vi "Process State Buffer.vi"(2 "AccelGyro constants":T3={"gyrRange"=0.0, "accRange"=0.0, "gx offset"=0.0, "gy offset"=0.0, "gz offset"=0.0, "ax offset"=0.0, "ay offset"=0.0, "az offset"=0.0, "axyz scale"=1.0} {"axyz scale" format="%#_4f"; "az offset" format="%#_4f"; "ay offset" format="%#_4f"; "ax offset" format="%#_4f"; "gz offset" format="%#_4f"; "gy offset" format="%#_4f"; "gx offset" format="%#_4f"; "gyrRange" format="%#_4f"; "accRange" format="%#_4f"}, 3 "STATE_Buffer excluding '$' [1...30]":string) -> (0 "Inertial state values":T2 {"w_z (dps)" format="%#_4f"; "a_y (g)" format="%#_4f"; "a_z (g)" format="%#_4f"; "w_y (dps)" format="%#_4f"; "a_x (g)" format="%#_4f"; "Sensor temp. (degC)" format="%#.2f"; "w_x (dps)" format="%#_4f"}, 1 "Environmental state values":T1 {"Dew point (degC)" format="%#.2f"; "Density (kg/m^3)" format="%#.3f"; "Pressure alt. (m)" format="%#.2f"; "Density alt. (m)" format="%#.2f"; "Rel. Humidity (%)" format="%#.2f"; "P_atmos (Pa)" format="%#_6f"; "Sensor temp. (degC)" format="%#.2f"; "Thermistor (degC)" format="%#.2f"})   [LabVIEW 2020]
uses:
  Ctls/AccelGyro constants.ctl
  Ctls/Inertial state values.ctl
  Ctls/Environmental state values.ctl
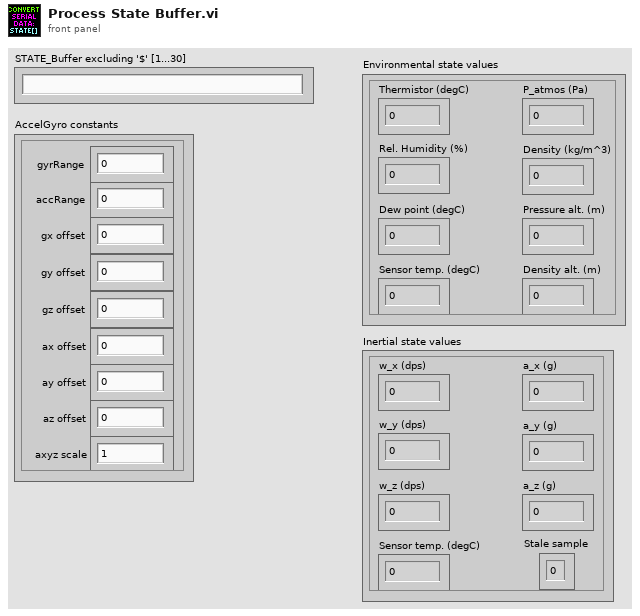
[diagram p1: front panel]
types:
  T1 = typedef "Environmental state values.ctl" = cluster{"Thermistor (degC)":sgl, "Sensor temp. (degC)":sgl, "P_atmos (Pa)":sgl, "Rel. Humidity (%)":sgl, "Density (kg/m^3)":sgl, "Dew point (degC)":sgl, "Pressure alt. (m)":sgl, "Density alt. (m)":sgl}
  T2 = typedef "Inertial state values.ctl" = cluster{"w_x (dps)":sgl, "w_y (dps)":sgl, "w_z (dps)":sgl, "a_x (g)":sgl, "a_y (g)":sgl, "a_z (g)":sgl, "Stale sample":u8, "Sensor temp. (degC)":sgl}
  T3 = typedef "AccelGyro constants.ctl" = cluster{"gyrRange":sgl, "accRange":sgl, "gx offset":sgl, "gy offset":sgl, "gz offset":sgl, "ax offset":sgl, "ay offset":sgl, "az offset":sgl, "axyz scale":sgl}
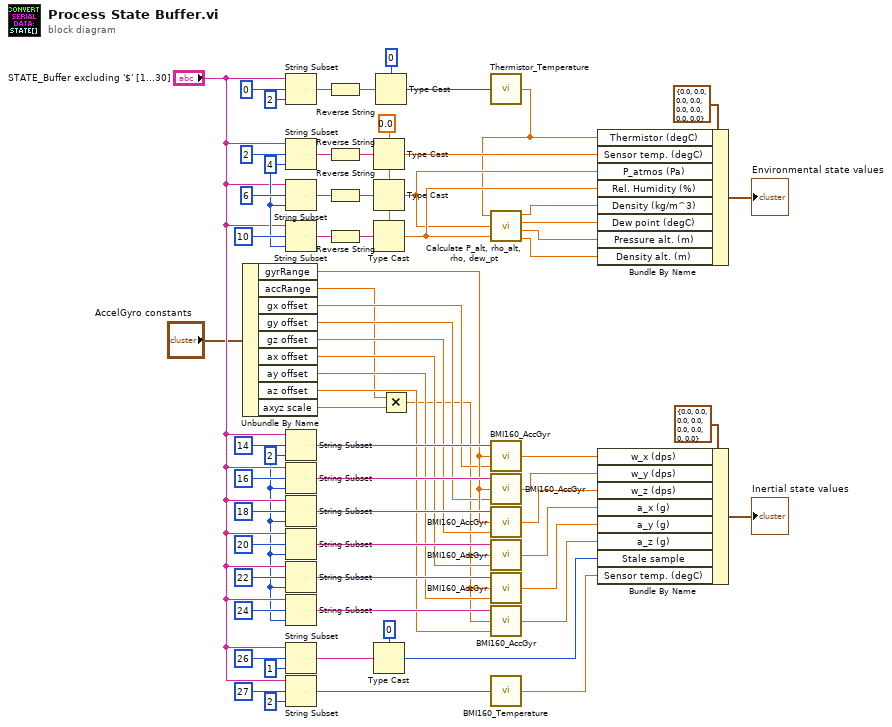
[diagram p0: block diagram]
diagram:
  w38 = 2 ("length (rest)")
  w58 = sgl 0.0
  w56 = 4 ("length (rest)")
  n1 = Unbundle By Name("AccelGyro constants") -> ("gyrRange"=w36:sgl, "accRange"=w28:sgl, "gx offset"=w35:sgl, "gy offset"=w34:sgl, "gz offset"=w33:sgl, "ax offset"=w32:sgl, "ay offset"=w31:sgl, "az offset"=w30:sgl, "axyz scale"=w29:sgl)
  n2 = String Subset(string="STATE_Buffer excluding '$' [1...30]", offset (0)=0, length (rest)=2 ("length (rest)")) -> (substring=w67:string)
  n3 = String Subset(string="STATE_Buffer excluding '$' [1...30]", offset (0)=2, length (rest)=w56) -> (substring=w63:string)
  n4 = String Subset(string="STATE_Buffer excluding '$' [1...30]", offset (0)=6, length (rest)=w56) -> (substring=w62:string)
  n5 = String Subset(string="STATE_Buffer excluding '$' [1...30]", offset (0)=10, length (rest)=w56) -> (substring=w59:string)
  n6 = String Subset(string="STATE_Buffer excluding '$' [1...30]", offset (0)=14, length (rest)=w38) -> (substring=w55:string)
  n7 = String Subset(string="STATE_Buffer excluding '$' [1...30]", offset (0)=16, length (rest)=w38) -> (substring=w54:string)
  n8 = String Subset(string="STATE_Buffer excluding '$' [1...30]", offset (0)=18, length (rest)=w38) -> (substring=w50:string)
  n9 = String Subset(string="STATE_Buffer excluding '$' [1...30]", offset (0)=20, length (rest)=w38) -> (substring=w51:string)
  n10 = String Subset(string="STATE_Buffer excluding '$' [1...30]", offset (0)=22, length (rest)=w38) -> (substring=w47:string)
  n11 = String Subset(string="STATE_Buffer excluding '$' [1...30]", offset (0)=24, length (rest)=w38) -> (substring=w46:string)
  n12 = String Subset(string="STATE_Buffer excluding '$' [1...30]", offset (0)=26, length (rest)=1 ("length (rest)")) -> (substring=w42:string)
  n13 = String Subset(string="STATE_Buffer excluding '$' [1...30]", offset (0)=27, length (rest)=2 ("length (rest)")) -> (substring=w37:string)
  n14 = Reverse String(1:w67) -> (0:w13:string)
  n15 = Reverse String(1:w63) -> (0:w12:string)
  n16 = Reverse String(1:w62) -> (0:w11:string)
  n17 = Reverse String(1:w59) -> (0:w10:string)
  n18 = Type Cast(type=w58, x=w12) -> (*(type *) &x=w3:sgl)
  n19 = Type Cast(type=w58, x=w11) -> (*(type *) &x=w4:sgl)
  n20 = Type Cast(type=w58, x=w10) -> (*(type *) &x=w5:sgl)
  n21 = Type Cast(type=u8 0, x=w42) -> (*(type *) &x=w17:u8)
  n22 = Type Cast(type=u16 0, x=w13) -> (*(type *) &x=w65:u16)
  n23 = Multiply(x=w28, y=w29) -> (x*y=w27:sgl)
  n24 = call "Thermistor_Temperature.vi"("T word"=w65) -> ("Temperature (degC)"=w2:sgl)
  n25 = call "Calculate P_alt, rho_alt, rho, dew_pt.vi"("Temperature (degC)"=w2, "Pressure (Pa)"=w4, "Rel. Hum. (%)"=w5) -> ("Density (kg/m^3)"=w6:sgl, "Dew point (degC)"=w7:sgl, "Pressure alt. (m)"=w8:sgl, "Density alt. (m)"=w9:sgl)
  n26 = call "BMI160_AccGyr.vi"("Offset"=w35, "Range"=w36, "Word (string, big endian)"=w55) -> ("eng val"=w23:sgl)
  n27 = call "BMI160_AccGyr.vi"("Offset"=w34, "Range"=w36, "Word (string, big endian)"=w54) -> ("eng val"=w22:sgl)
  n28 = call "BMI160_AccGyr.vi"("Offset"=w33, "Range"=w36, "Word (string, big endian)"=w50) -> ("eng val"=w21:sgl)
  n29 = call "BMI160_AccGyr.vi"("Offset"=w32, "Range"=w27, "Word (string, big endian)"=w51) -> ("eng val"=w20:sgl)
  n30 = call "BMI160_AccGyr.vi"("Offset"=w31, "Range"=w27, "Word (string, big endian)"=w47) -> ("eng val"=w19:sgl)
  n31 = call "BMI160_AccGyr.vi"("Offset"=w30, "Range"=w27, "Word (string, big endian)"=w46) -> ("eng val"=w18:sgl)
  n32 = call "BMI160_Temperature.vi"("Word (string, big endian)"=w37) -> ("T (deg C)"=w16:sgl)
  n33 = Bundle By Name(cluster=T1 {"Thermistor (degC)"=0.0, "Sensor temp. (degC)"=0.0, "P_atmos (Pa)"=0.0, "Rel. Humidity (%)"=0.0, "Density (kg/m^3)"=0.0, "Dew point (degC)"=0.0, "Pressure alt. (m)"=0.0, "Density alt. (m)"=0.0} ("Environmental state values"), "Thermistor (degC)"=w2, "Sensor temp. (degC)"=w3, "P_atmos (Pa)"=w4, "Rel. Humidity (%)"=w5, "Density (kg/m^3)"=w6, "Dew point (degC)"=w7, "Pressure alt. (m)"=w8, "Density alt. (m)"=w9) -> (→"Environmental state values":T1)
  n34 = Bundle By Name(cluster=T2 {"w_x (dps)"=0.0, "w_y (dps)"=0.0, "w_z (dps)"=0.0, "a_x (g)"=0.0, "a_y (g)"=0.0, "a_z (g)"=0.0, "Stale sample"=0, "Sensor temp. (degC)"=0.0} ("Environmental state values"), "w_x (dps)"=w23, "w_y (dps)"=w22, "w_z (dps)"=w21, "a_x (g)"=w20, "a_y (g)"=w19, "a_z (g)"=w18, "Stale sample"=w17, "Sensor temp. (degC)"=w16) -> (→"Inertial state values":T2)
